vi "Execute Prepared SQL (string results).vi"(8 "error in (no error)":errorcluster, 11 "SQL Statement in":refnum<class "SQL Statement.lvclass">) -> (0 "error out":errorcluster, 2 "Result Set":string[][](array[string]), 3 "SQL Statement out":refnum<class "SQL Statement.lvclass">)   [LabVIEW 2011, in "SQLite.lvlib" / "SQL Statement.lvclass"]
uses:
  SQL Statement.lvclass
  SQL Statement.lvclass/SQL Statement.ctl
  Error Message.vi
  Column String.vi
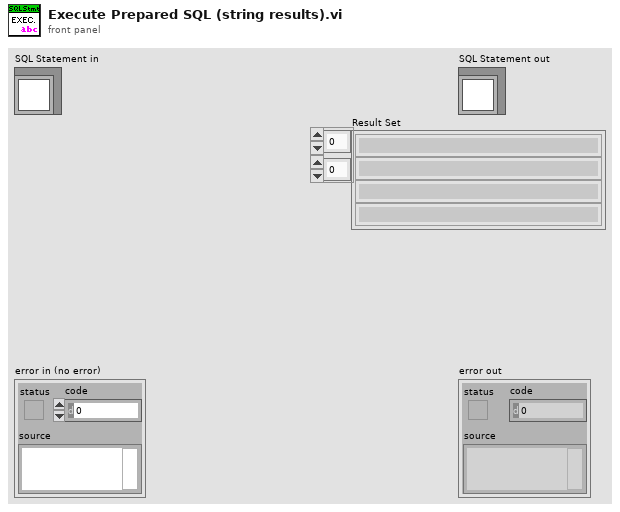
[diagram p1: front panel]
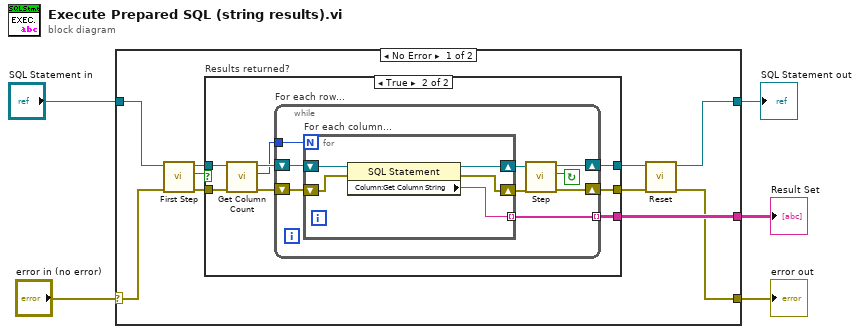
[diagram p0: block diagram]
diagram:
  n1 = case shown="No Error" "error in (no error)" {
    selector: "error in (no error)" -> [w11 w41]
    tunnel: [w13 w41] -> w3
    tunnel: [w14 w40] -> w1
    tunnel: "SQL Statement in" -> [w12 w40]
    tunnel: [w15 _] -> w2
    frame No Error {
      n2 = call "First Step.vi"("error in (no error)"=w11, "SQL Statement in"=w12) -> ("error out"=w9:errorcluster, "Row returned"=w8:bool, "SQL Statement out"=w10:refnum<class "SQL Statement.lvclass">)  [unwired: 7 in]
      n3 = case "Results returned?" shown="True" w8 {
        tunnel: [w17 w25] -> w7
        tunnel: [w16 w24] -> w6
        tunnel: w10 -> [w17 w23]
        tunnel: w9 -> [w16 w19]
        tunnel: [_ w22] -> w15
        frame False {
        }
        frame True {
          n4 = call "Get Column Count.vi"("error in (no error)"=w19, "SQL Statement in"=w23) -> ("error out"=w18:errorcluster, "Number of Columns"=w20:i32, "SQL Statement out"=w21:refnum<class "SQL Statement.lvclass">)  [unwired: 7 in]
          n5 = while "For each row..." {
            shift-right: [w33] -> w25
            shift-left: w21 -> [w30]
            shift-right: [w31] -> w24
            shift-left: w18 -> [w29]
            tunnel: [w28] -> w22 mode=indexing
            tunnel: w20 -> [w26]
            stop <- w27 continue-if-true
            n6 = for "For each column..." {
              N: w26 -> [_]
              tunnel: [w35] -> w28 mode=indexing
              shift-right: [w36] -> w34
              shift-left: w30 -> [w39]
              shift-right: [w37] -> w32
              shift-left: w29 -> [w38]
              n7 = property class="SQL Statement"(reference=w39, error in=w38) -> (reference out=w36:refnum<class "SQL Statement.lvclass">, error out=w37:errorcluster, "Column:Get Column String"=w35:string)
            }
            n8 = call "Step.vi"("error in (no error)"=w32, "SQL Statement in"=w34) -> ("error out"=w31:errorcluster, "Row returned"=w27:bool, "SQL Statement out"=w33:refnum<class "SQL Statement.lvclass">)  [unwired: 7 in]
          }
        }
      }
      n9 = call "Reset.vi"("error in (no error)"=w6, "SQL Statement in"=w7) -> ("error out"=w13:errorcluster, "SQL Statement out"=w14:refnum<class "SQL Statement.lvclass">)  [unwired: 8 in]
    }
    frame Error {
    }
  }
  "error out" <- w3
  "SQL Statement out" <- w1
  "Result Set" <- w2
